vi "Encoder Position & Velocity (Host).vi"() -> ()   [LabVIEW 2009]
doc: "Real Time Host vi for Quadrature Encoder Velocity and Acceleration Estimation using CompactRIO.\n\nThis application is designed to work with an R-Series expansion setup using FPGA-7811R and a CompactRIO cRIO-9411 digital input module installed in slot 1 of the expansion chassis.\n\nBefore Executing the vi:\n1. Select the FPGA Resource in the VISA Resource Name Control\n2. Specify a Fixed Time Interval for Velocity and Acceleration Estimation\n3. Specify the Pulses/revolution for the Quadrature Encoder\n4. Run the vi"
uses:
  <vilib>/userDefined/High Color/nirio_resource_hc.ctl
  <vilib>/rvi/interface/nirviOpenFPGA/nirviOpenFPGA.xnode
  FPGA Bitfiles/Q_IGVC_2010.lvproj_FPGA Target_FPGA_MAIN.vi.lvbitx
  <vilib>/FPGAPlugInAG/cRIO-9113/nirviIntfOpen_cRIO-9113.vi
  <vilib>/rvi/interface/nirviReadWriteControl/nirviReadWriteControl.xnode
  <vilib>/Utility/error.llb/Error Cluster From Error Code.vi
  <vilib>/rvi/errors/niLvFpgaAdjustHostInterfaceError.vi
  <vilib>/rvi/interface/common/niFpgaNodeNameForErrorReporting.ctl
  <vilib>/rvi/errors/niLvFpgaWhatHappensToTopLevelVI.ctl
  <vilib>/rvi/interface/nirviCloseFPGA/nirviCloseFPGA.xnode
  <vilib>/FPGAPlugInAG/cRIO-9113/nirviIntfClose_cRIO-9113.vi
  NiRioSrv.dll
panel:
  in  "stop":bool
  out "Left Dist. Travelled (Cm)":dbl
  out "Right Dist. Travelled (Cm)":dbl
  out "Left Acceleration (rps/s)":dbl
  out "Left Velocity (RPM)":dbl
  out "Right Acceleration (rps/s)":dbl
  out "Right Velocity (RPM)":dbl
  out "Left Position (Counts)":i32
  out "Right Position (Counts)":i32
  in  "Pulses/Revolution":i32=2000
  in  "Fixed Time \nInterval (uSec)":u32=1000
  in  "Reset Position":bool
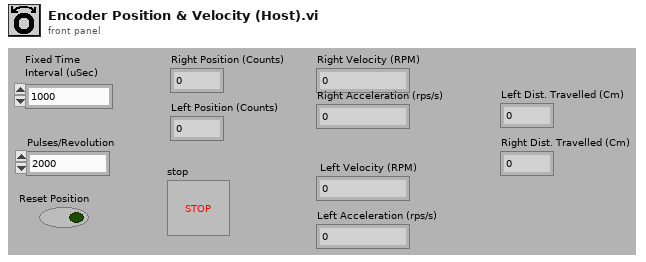
[diagram p1: front panel]
types:
  T1 = typedef "nirio_resource_hc.ctl" = tag
  T2 = typedef "niFpgaNodeNameForErrorReporting.ctl" = enum16{"Open FPGA VI Reference", "Read/Write Control", "Invoke Method: Abort", "Invoke Method: Acknowledge IRQ", "Invoke Method: Download", "Invoke Method: FIFO.Configure", "Invoke Method: FIFO.Read", "Invoke Method: FIFO.Start", "Invoke Method: FIFO.Stop", "Invoke Method: FIFO.Write", "Invoke Method: Reset", "Invoke Method: Run", "Invoke Method: Wait on IRQ", "Close FPGA VI Reference"}
  T3 = typedef "niLvFpgaWhatHappensToTopLevelVI.ctl" = enum16{"top level VI scripted behind XNode", "top level VI inlined behind XNode"}
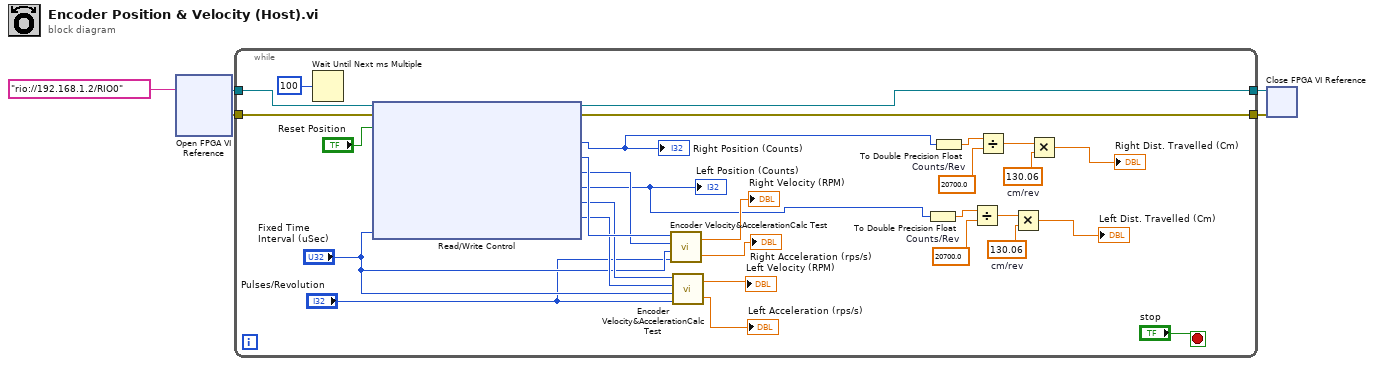
[diagram p0: block diagram]
diagram:
  n1 = xnode "Open FPGA VI Reference"("resource name"=T1 "rio://192.168.1.2/RIO0") -> ("FPGA VI Reference Out"=w5:refnum<k20>, "error out"=w3:errorcluster)  [unwired: 1 in]
  n2 = while {
    tunnel: w5 -> [w34]
    tunnel: [w33] -> w4
    tunnel: w3 -> [w31]
    tunnel: [w30] -> w2
    stop <- "stop" stop-if-true
    w9 = 130.06  # cm/rev
    w11 = 130.06  # cm/rev
    w14 = 20700.0  # Counts/Rev
    w17 = 20700.0  # Counts/Rev
    n3 = Wait Until Next ms Multiple(millisecond multiple=u32 100) -> ()  [unwired: 1 out]
    n4 = xnode "Read/Write Control"("FPGA VI Reference In"=w34, "error in"=w31, "Position Reset"="Reset Position", "Velocity Interval (uSec)"="Fixed Time \nInterval (uSec)") -> ("FPGA VI Reference Out"=w33:refnum<k20>, "error out"=w30:errorcluster, "Right Position (Counts)"=w16:i32, "Right Velocity (Counts/Interval)"=w29:i32, "Right Acceleration (Counts/Interval)"=w27:i32, "Left Position (Counts)"=w13:i32, "Left Velocity (Counts/Interval)"=w26:i32, "Left Acceleration (Counts/Interval)"=w25:i32)
    "Right Position (Counts)" <- w16
    "Left Position (Counts)" <- w13
    n5 = call "Encoder Velocity&AccelerationCalc Test.vi"("Pulses/Revolution"="Pulses/Revolution", "Fixed Time \nInterval (uSec)"="Fixed Time \nInterval (uSec)", "Acceleration (Counts/Interval)"=w27, "Velocity (Counts/Interval)"=w29) -> ("Acceleration (rps/s)"=→"Right Acceleration (rps/s)":dbl, "Velocity (RPM)"=→"Right Velocity (RPM)":dbl)
    n6 = call "Encoder Velocity&AccelerationCalc Test.vi"("Pulses/Revolution"="Pulses/Revolution", "Fixed Time \nInterval (uSec)"="Fixed Time \nInterval (uSec)", "Acceleration (Counts/Interval)"=w25, "Velocity (Counts/Interval)"=w26) -> ("Acceleration (rps/s)"=→"Left Acceleration (rps/s)":dbl, "Velocity (RPM)"=→"Left Velocity (RPM)":dbl)
    n7 = To Double Precision Float(number=w13) -> (double precision float=w15:dbl)
    n8 = To Double Precision Float(number=w16) -> (double precision float=w18:dbl)
    n9 = Divide(x=w15, y=w14) -> (x/y=w7:dbl)
    n10 = Divide(x=w18, y=w17) -> (x/y=w12:dbl)
    n11 = Multiply(x=w7, y=w9) -> (x*y=→"Left Dist. Travelled (Cm)":dbl)
    n12 = Multiply(x=w12, y=w11) -> (x*y=→"Right Dist. Travelled (Cm)":dbl)
  }
  n13 = xnode "Close FPGA VI Reference"("FPGA VI Reference In"=w4, "error in"=w2) -> ()  [unwired: 1 out]
